vi "brojac_tajmer.vi"() -> ()   [LabVIEW 2023]
uses:
  enum_kontrola_vjezbe.ctl
panel:
  out "error out":errorcluster
  in  "error in (no error)":errorcluster
  out "Numeric":dbl
  in  "Enum":T1
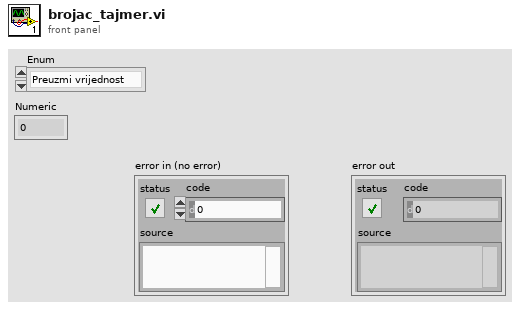
[diagram p1: front panel]
types:
  T1 = typedef "enum_kontrola_vjezbe.ctl" = enum16{"Preuzmi vrijednost", "Ponisti", "Povecaj", "Smanji"}
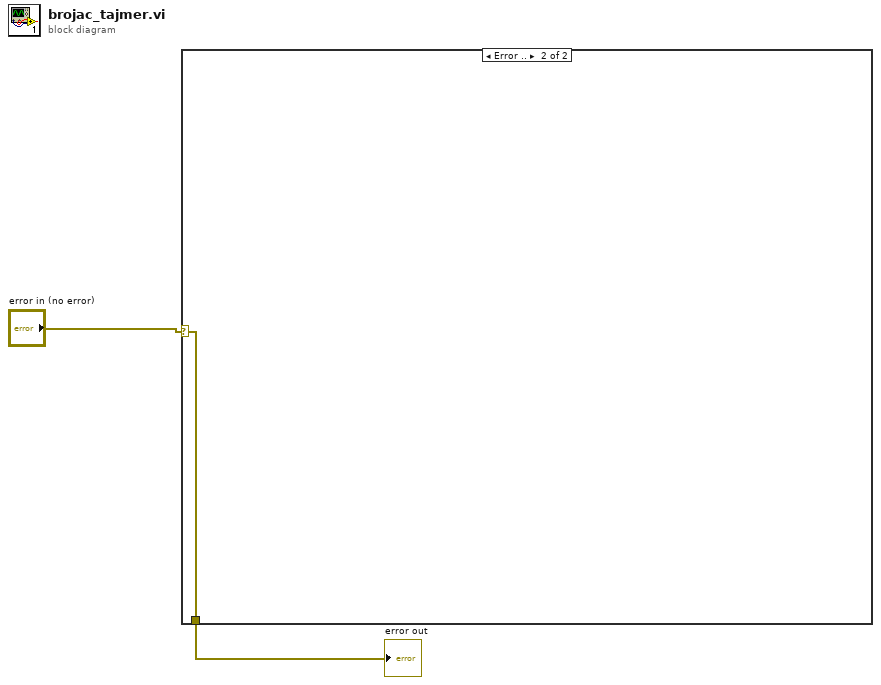
[diagram p0: block diagram]
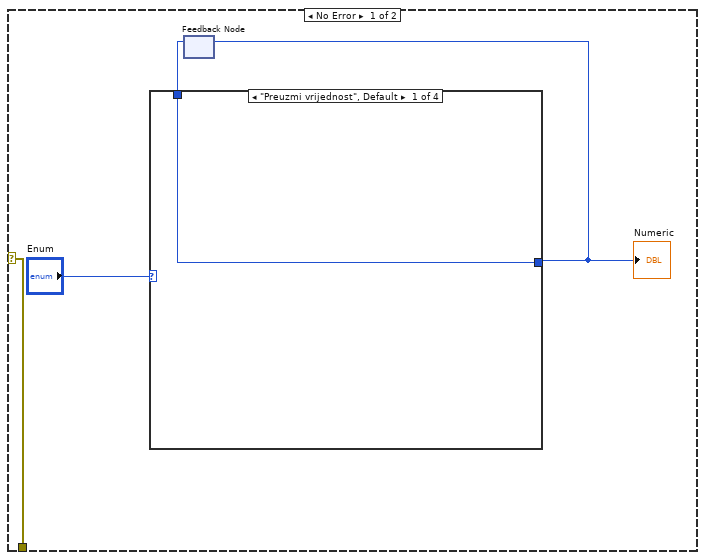
[diagram p2: hidden frame]
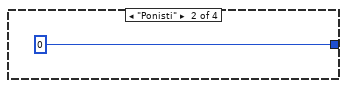
[diagram p3: hidden frame]
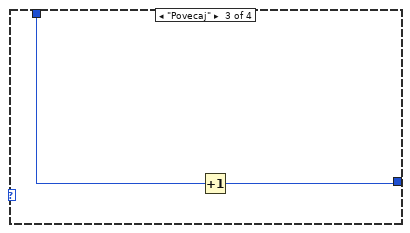
[diagram p4: hidden frame]
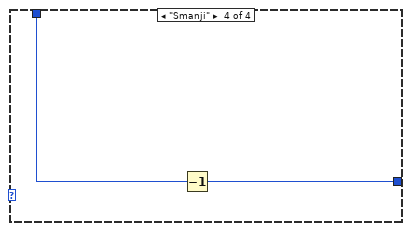
[diagram p5: hidden frame]
diagram:
  n1 = case shown="Error .." "error in (no error)" {
    selector: "error in (no error)" -> [w3 w13]
    tunnel: [w3 w13] -> w1
    frame No Error {
      n2 = feedback #1() -> (w4:i32)  [unwired: 1 in]
      n3 = case shown="\"Preuzmi vrijednost\", Default" "Enum" {
        tunnel: [w7 0 w9 w12] -> w5
        tunnel: w4 -> [w7 _ w10 w11]
        frame "Preuzmi vrijednost", Default {
        }
        frame "Ponisti" {
        }
        frame "Povecaj" {
          n4 = Increment(x=w10) -> (x+1=w9:i32)
        }
        frame "Smanji" {
          n5 = Decrement(x=w11) -> (x-1=w12:i32)
        }
      }
      "Numeric" <- w5
      n6 = feedback-in #1(w5) -> ()
    }
    frame Error {
    }
  }
  "error out" <- w1
